vi "Main_EEG Tab_Control.vi"() -> ()   [LabVIEW 2023]
panel:
  in  "Tab Control":T1(tab)
  in  "File Path":path
  out "Experiment Name":string
  out "Session Name":string
  out "Dataset\nof EEGs":dbl[][](array[numeric])
  out "Header\nof EEGs":string[](array[string])
  out "Representation of the EEG Signals":dbl[][](graph)
  in  "Sampling Frequency\nfor  Bandpass Filtering":dbl=200.0
  in  "Higher Cut-Off\nfor Highpass Filter":dbl=1.0
  in  "Lower Cut-Off\nfor Lowpass Filter":dbl=70.0
  in  "Absolute\nData":bool
  out "Denoised EEG Signals":dbl[][](graph)
  in  "Statistical Storement?":bool
  in  "Frequency Saver?":bool
  in  "Attribute Selection":u16(ring) items=["Periferal", "Central", "Frontal", "Temporal"]
  in  "Normalize Data?":bool
  out "Attribute Output":u16(ring) items=["Periferal", "Central", "Frontal", "Temporal"]
  out "Normalized EEG Signals":dbl[](graph)
  in  "Threshold\nPercentage":dbl=0.05
  in  "FFT Size":i32=3072000
  in  "Threshold Factor":dbl=10.0
  in  "FFT Factor":i32=16
  in  "Segment Partition":i32=10
  out "Dominant Frequencies":dbl[](array[numeric])
  in  "WaveletType":string="db04"
  in  "Levels":dbl=5.0
  out "Frequency Array":dbl[](array[numeric])
  out "Detected Wave":string
  out "Dominant Frequency\nin Wave (Hz)":dbl
  out "Detected Wave":string
  out "Dominant Frequency (Hz)":dbl
  out "FFT Wave Array":string[](array[string])
  out "MRA Wave Array":string[](array[string])
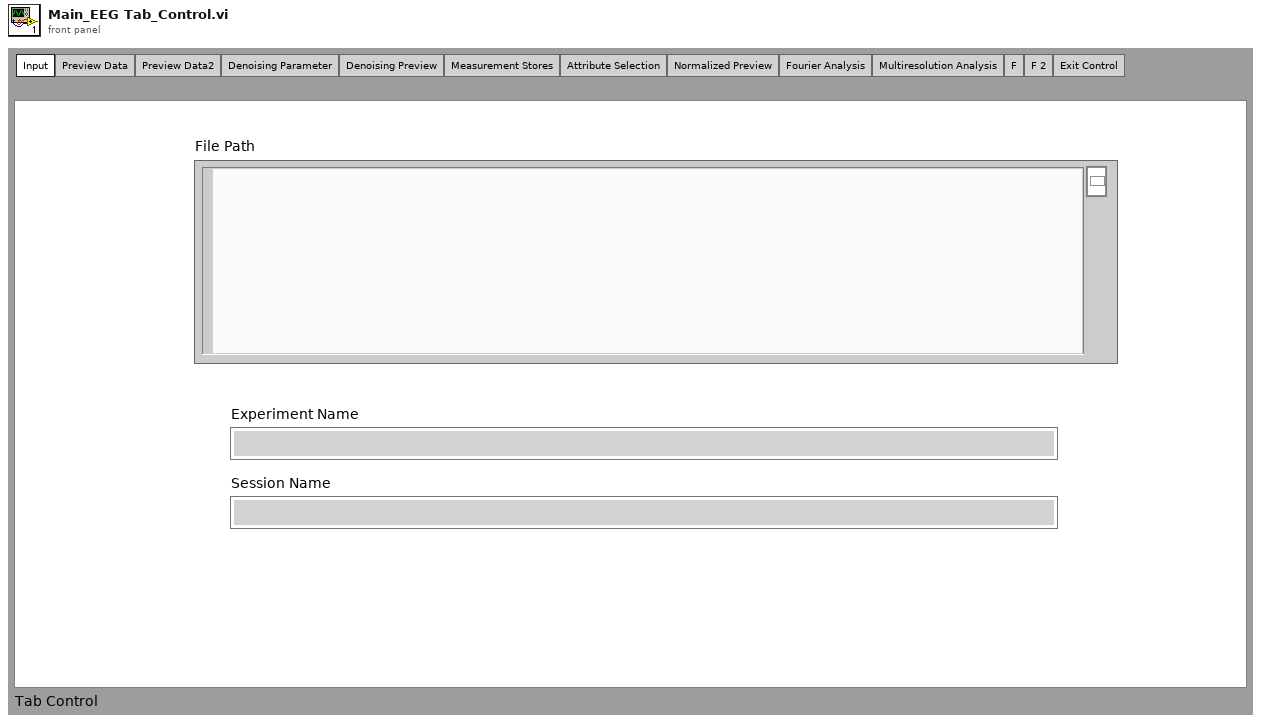
[diagram p1: front panel]
types:
  T1 = enum32{"Input", "Preview Data", "Preview Data2", "Denoising Parameter", "Denoising Preview", "Measurement Stores", "Attribute Selection", "Normalized Preview", "Fourier Analysis", "Multiresolution Analysis", "F", "F 2", "Exit Control"}
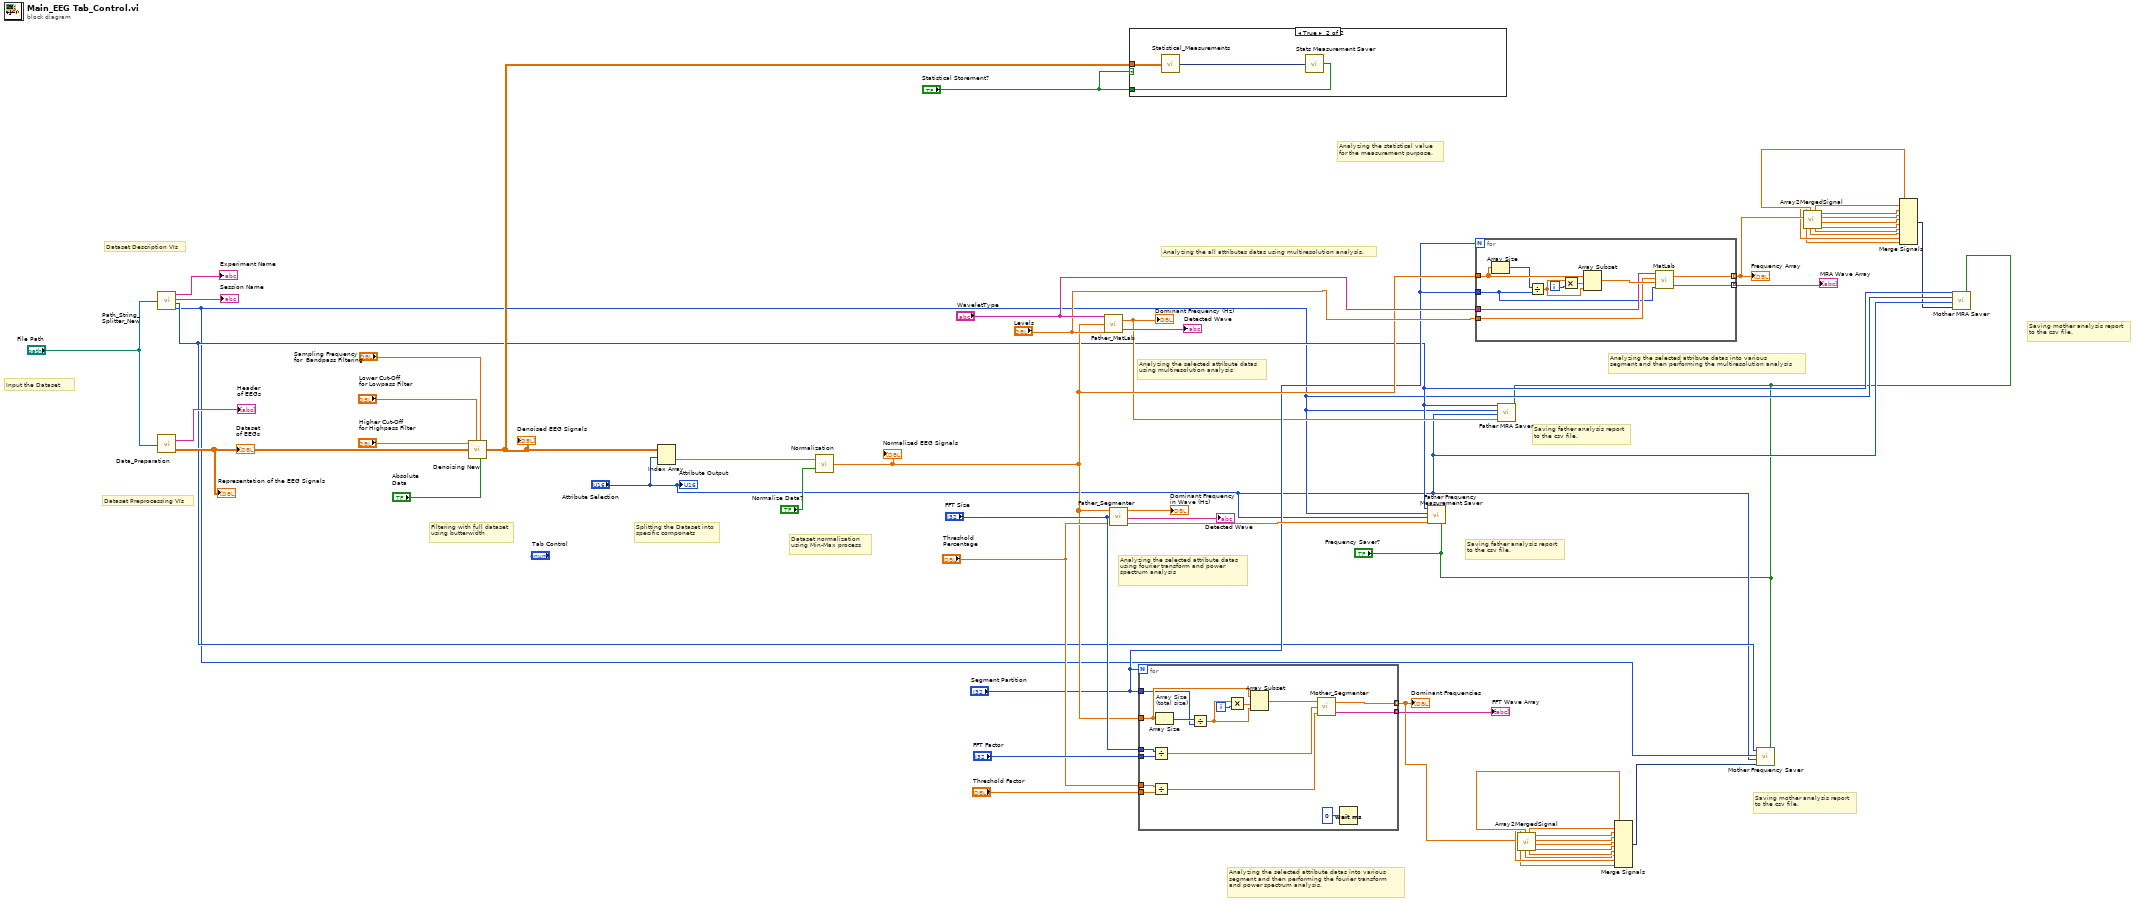
[diagram p0: block diagram]
diagram:
  # "Saving father analysis report\nto the csv file."
  # "Saving mother analysis report\nto the csv file."
  # "Analyzing the selected attribute datas into various\nsegment and then performing the multiresolution analysis"
  # "Analyzing the statistical value \nfor the measurement purpose."
  # "Analyzing the all attributes datas using multiresolution analysis."
  # "Analyzing the selected attribute datas\nusing multiresolution analysis"
  # "Saving mother analysis report\nto the csv file."
  # "Saving father analysis report\nto the csv file."
  # "Analyzing the selected attribute datas into various\nsegment and then performing the fourier transform\nand power spectrum analysis."
  # "Analyzing the selected attribute datas\nusing fourier transform and power \nspectrum analysis"
  # "Dataset normalization\nusing Min-Max process"
  # "Splitting the Dataset into\nspecific componets"
  # "Filtering with full dataset\nusing butterwidth"
  # "Dataset Preprocessing VIs"
  # "Dataset Description VIs"
  # "Input the Dataset"
  n1 = call "Path_String_Splitter_New.vi"("File Path"="File Path") -> ("Experiment Name"=→"Experiment Name":string, "Session Name"=→"Session Name":string, "Experment Index"=w29:i32, "Session Index"=w28:i32)
  n2 = call "Data_Preparation.vi"("File Path"="File Path") -> ("Header"=→"Header\nof EEGs":string[], "Datas"=w41:dbl[][])
  "Dataset\nof EEGs" <- w41
  "Representation of the EEG Signals" <- w41
  n3 = call "Denoising New.vi"("Higher Cut-Off\nfor Highpass Filter"="Higher Cut-Off\nfor Highpass Filter", "Lower Cut-Off\nfor Lowpass Filter"="Lower Cut-Off\nfor Lowpass Filter", "Array in"=w41, "Sampling Frequency\nfor  Bandpass Filtering"="Sampling Frequency\nfor  Bandpass Filtering", "Absolute Data"="Absolute\nData") -> ("Array out"=w42:dbl[][])  [unwired: 4 in]
  "Denoised EEG Signals" <- w42
  n4 = Index Array "Index Array"(array=w42, index (row)="Attribute Selection") -> (element=w51:dbl[])  [unwired: 1 in]
  n5 = call "Normalization.vi"("Normalize Data"="Normalize Data?", "Array in"=w51) -> ("Array out"=w33:dbl[])
  "Normalized EEG Signals" <- w33
  n6 = call "Father_MatLab.vi"("Levels"="Levels", "input Array"=w33, "WaveletType"="WaveletType") -> ("Detected Wave"=→"Detected Wave":string, "dominantFrequency"=w30:dbl)
  "Dominant Frequency (Hz)" <- w30
  n7 = call "Father_Segmenter.vi"("Threshold Percentage"="Threshold\nPercentage", "FFT Size"="FFT Size", "Array in"=w33) -> ("Merge Signals"=w37:dbl, "Detected Wave"=→"Detected Wave":string, "Dominant Frequency\nin Wave (Hz)"=→"Dominant Frequency\nin Wave (Hz)":dbl)
  n8 = case shown="True" "Statistical Storement?" {
    tunnel: w42 -> [_ w59]
    tunnel: "Statistical Storement?" -> [_ w57]
    frame False {
    }
    frame True {
      n9 = call "Statistical_Measurements.vi"("Array"=w59) -> ("Dynamic Data"=w58:dynamicdata)
      n10 = call "Stats Measurement Saver.vi"("Dynamic Data"=w58, "OK Button"=w57) -> ()
    }
  }
  n11 = for {
    N: "Segment Partition" -> [_]
    tunnel: w33 -> [w67]
    tunnel: "Segment Partition" -> [w65]
    tunnel: "FFT Size" -> [w73]
    tunnel: "FFT Factor" -> [w71]
    tunnel: "Threshold\nPercentage" -> [w69]
    tunnel: "Threshold Factor" -> [w68]
    tunnel: [w60] -> w2 mode=indexing
    tunnel: [w62] -> w38 mode=indexing
    i -> [w61]
    n12 = Divide(x=w73, y=w71) -> (x/y=w72:dbl)
    n13 = Divide(x=w69, y=w68) -> (x/y=w70:dbl)
    n14 = Array Size "Array Size\n(total size)"(array=w67) -> (size(s)=w75:i32)
    n15 = Divide(x=w75, y=w65) -> (x/y=w63:dbl)
    n16 = Multiply(x=w63, y=w61) -> (x*y=w66:dbl)
    n17 = Array Subset "Array Subset"(array=w67, index=w66, length=w63) -> (w74:dbl[])
    n18 = call "Mother_Segmenter.vi"("Threshold Percentage"=w70, "FFT Size"=w72, "Array in"=w74) -> ("Detected Wave"=w62:string, "Dominant Frequency\nin Wave (Hz)"=w60:dbl)
    n19 = Wait (ms)(milliseconds to wait=u32 0) -> ()  [unwired: 1 out]
  }
  "Dominant Frequencies" <- w2
  "FFT Wave Array" <- w38
  n20 = call "Father Frequency Measurement Saver.vi"("Frequency Saver?"="Frequency Saver?", "Dynamic Data"=w37, "Feature Index"="Attribute Selection", "Session Index"=w28, "Experiment Index"=w29) -> ()
  n21 = for {
    N: "Segment Partition" -> [_]
    tunnel: w33 -> [w85]
    tunnel: "Segment Partition" -> [w76]
    tunnel: "WaveletType" -> [w80]
    tunnel: "Levels" -> [w79]
    tunnel: [w78] -> w24 mode=indexing
    tunnel: [w77] -> w31 mode=indexing
    i -> [w86]
    n22 = Array Size(array=w85) -> (size(s)=w82:i32)
    n23 = Divide(x=w82, y=w76) -> (x/y=w83:dbl)
    n24 = Multiply(x=w83, y=w86) -> (x*y=w84:dbl)
    n25 = Array Subset "Array Subset"(array=w85, index=w84, length=w83) -> (w81:dbl[])
    n26 = call "MatLab.vi"("Segment"=w76, "input Array"=w81, "Levels"=w79, "WaveletType"=w80) -> ("Detected Wave"=w77:string, "dominantFrequency"=w78:dbl)
  }
  "Frequency Array" <- w24
  "MRA Wave Array" <- w31
  n27 = call "Father MRA Saver.vi"("Frequency Saver?"="Frequency Saver?", "Dynamic Data"=w30, "Feature Index"="Attribute Selection", "Session Index"=w28, "Experiment Index"=w29) -> ()
  n28 = call "Array2MergedSignal.vi"("Array"=w2) -> ("Dynamic Data Type 6"=w7:dbl, "Dynamic Data Type 5"=w8:dbl, "Dynamic Data Type 4"=w9:dbl, "Dynamic Data Type 3"=w10:dbl, "Dynamic Data Type 7"=w6:dbl, "Dynamic Data Type 2"=w11:dbl, "Dynamic Data Type 8"=w5:dbl, "Dynamic Data Type"=w12:dbl, "Dynamic Data Type 10"=w3:dbl, "Dynamic Data Type 9"=w4:dbl)  [unwired: 1 in]
  n29 = Merge Signals(w12, w11, w10, w9, w8, w7, w6, w5, w4, w3) -> (w1:dynamicdata)
  n30 = call "Mother Frequency Saver.vi"("Frequency Saver?"="Frequency Saver?", "Dynamic Data"=w1, "Feature Index"="Attribute Selection", "Session Index"=w28, "Experiment Index"=w29) -> ()
  n31 = call "Array2MergedSignal.vi"("Array"=w24) -> ("Dynamic Data Type 6"=w18:dbl, "Dynamic Data Type 5"=w19:dbl, "Dynamic Data Type 4"=w20:dbl, "Dynamic Data Type 3"=w21:dbl, "Dynamic Data Type 7"=w17:dbl, "Dynamic Data Type 2"=w22:dbl, "Dynamic Data Type 8"=w16:dbl, "Dynamic Data Type"=w23:dbl, "Dynamic Data Type 10"=w14:dbl, "Dynamic Data Type 9"=w15:dbl)  [unwired: 1 in]
  n32 = Merge Signals(w23, w22, w21, w20, w19, w18, w17, w16, w15, w14) -> (w13:dynamicdata)
  n33 = call "Mother MRA Saver.vi"("Frequency Saver?"="Frequency Saver?", "Dynamic Data"=w13, "Feature Index"="Attribute Selection", "Session Index"=w28, "Experiment Index"=w29) -> ()
  "Attribute Output" <- "Attribute Selection"
